vi "createInboundChannel.vi"(8 "error in (no error)":errorcluster, 11 "Connection.NetworkStream in":refnum<class "Connection.NetworkStream.lvclass">) -> (0 "error out":errorcluster, 2 "Authorization":T1, 3 "Connection.NetworkStream out":refnum<class "Connection.NetworkStream.lvclass">)   [LabVIEW 2013, in "Connection.NetworkQueue_GOSPL.lvlib" / "Connection.NetworkStream.lvclass"]
uses:
  Connection.NetworkStream.lvclass
  Connection/auth -- cluster.ctl
  Connection.NetworkStream.lvclass/Connection.NetworkStream.ctl
  Connection/Connection.lvclass
  Connection/Connection.lvclass/Connection.ctl
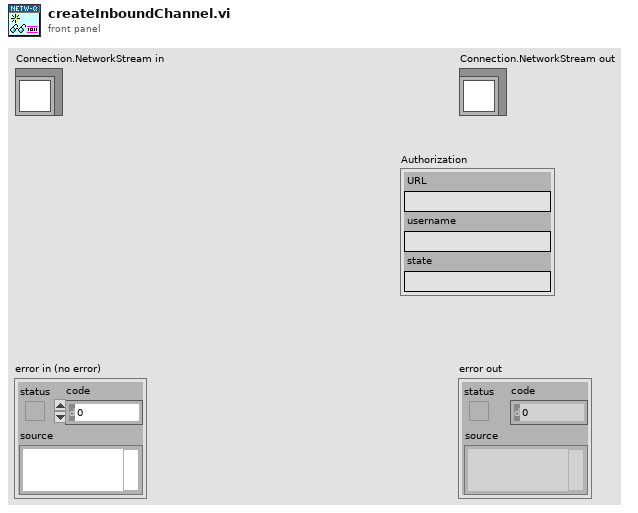
[diagram p1: front panel]
types:
  T1 = typedef "Connection_GOSPL.lvlib/Connection.lvclass/auth -- cluster.ctl" = cluster{"URL":string, "username":string, "state":string}
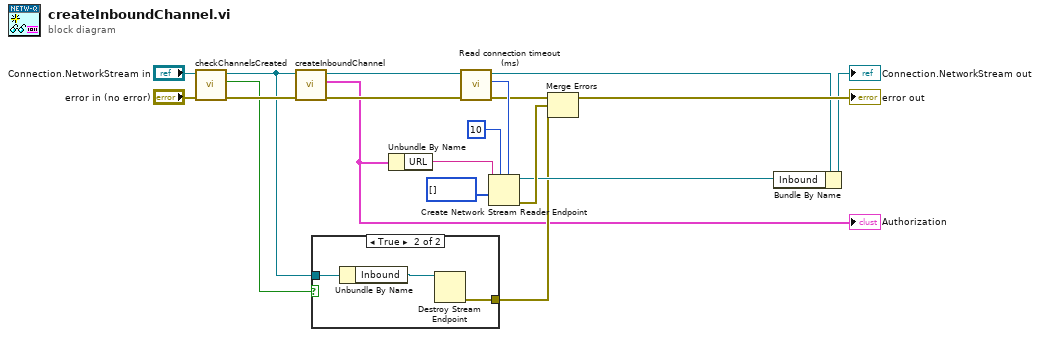
[diagram p0: block diagram]
diagram:
  n1 = call-dynamic "checkChannelsCreated.vi"("error in (no error)"="error in (no error)", "Connection.NetworkStream in"="Connection.NetworkStream in") -> ("error out"=w7:errorcluster, "inbound created"=w6:bool, "Connection.NetworkStream out"=w5:refnum<class "Connection.NetworkStream.lvclass">)  [unwired: 6 in, 1 out]
  n2 = call-parent "createInboundChannel.vi"("error in (no error)"=w7, "Connection in"=w5) -> ("error out"=w16:errorcluster, "Authorization"=w1:T1, "Connection out"=w3:refnum<class "Connection.NetworkStream.lvclass">)  [unwired: 7 in]
  "Authorization" <- w1
  n3 = case shown="True" w6 {
    tunnel: w5 -> [_ w22]
    tunnel: [_ w20] -> w4
    frame False {
    }
    frame True {
      n4 = Unbundle By Name(w22) -> ("Inbound"=w21:refnum<k21>)
      n5 = Destroy Stream Endpoint(11:w21) -> (0:w20:errorcluster)  [unwired: 1 in]
    }
  }
  n6 = Unbundle By Name(w1) -> ("URL"=w2:string)
  n7 = call "Read connection timeout (ms).vi"("error in (no error)"=w16, "Connection in"=w3) -> ("error out"=w14:errorcluster, "connection timeout (ms)"=w17:i32, "Connection out"=w11:refnum<class "Connection.NetworkStream.lvclass">)  [unwired: 7 in]
  n8 = Create Network Stream Reader Endpoint(5:w17, 7:10 ("reader buffer size"), 9:u8[] [] ("Bytes Stream"), 11:w2) -> (0:w15:errorcluster, 3:w12:refnum<k21>)  [unwired: 3 in]
  n9 = Merge Errors(w14, w15, w4) -> (→"error out":errorcluster)
  n10 = Bundle By Name(cluster=w11, "Inbound"=w12) -> (→"Connection.NetworkStream out":refnum<class "Connection.NetworkStream.lvclass">)
